vi "Build-Get Specs.vi"() -> (4 "project":refnum<vi>, 6 "specs":refnum<vi>[](array[refnum]), 15 "error out":errorcluster)   [LabVIEW 2020]
panel:
  out "Path":path
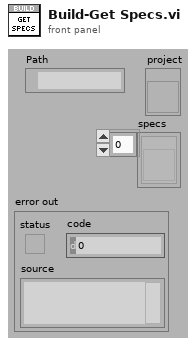
[diagram p1: front panel]
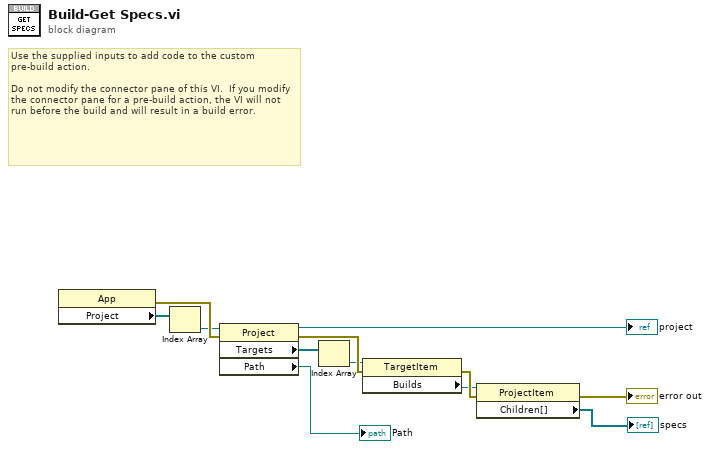
[diagram p0: block diagram]
diagram:
  # "Use the supplied inputs to add code to the custom pre-build action.\n\nDo not modify the connector pane of this VI.  If you modify the connector pane for a pre-build action, the VI will not run before the build and will result in a build error."
  n1 = property class="App"() -> (error out=w12:errorcluster, "Project"=w9:refnum<vi>[])  [unwired: 2 in, 1 out]
  n2 = Index Array(array=w9) -> (element=w8:refnum<vi>)  [unwired: 1 in]
  n3 = property class="Project"(reference=w8, error in=w12) -> (reference out=→"project":refnum<vi>, error out=w11:errorcluster, "Targets"=w7:refnum<vi>[], "Path"=→"Path":path)
  n4 = Index Array(array=w7) -> (element=w6:refnum<vi>)  [unwired: 1 in]
  n5 = property class="TargetItem"(reference=w6, error in=w11) -> (error out=w10:errorcluster, "Builds"=w5:refnum<vi>)  [unwired: 1 out]
  n6 = property class="ProjectItem"(reference=w5, error in=w10) -> (error out=→"error out":errorcluster, "Children[]"=→"specs":refnum<vi>[])  [unwired: 1 out]
